vi "Digital Input Data.vi"(8 "error in (no error)":errorcluster, 10 "Digital Input Data":bool[](array[boolean]), 11 "Digital Reader in":refnum<class "Digital Reader.lvclass">) -> (0 "error out":errorcluster, 3 "Digital Reader out":refnum<class "Digital Reader.lvclass">)   [LabVIEW 2024, in "DAQmx Actor.lvlib" / "Digital Reader.lvclass"]
uses:
  Digital Reader.lvclass
  Digital Reader.lvclass/Digital Reader.ctl
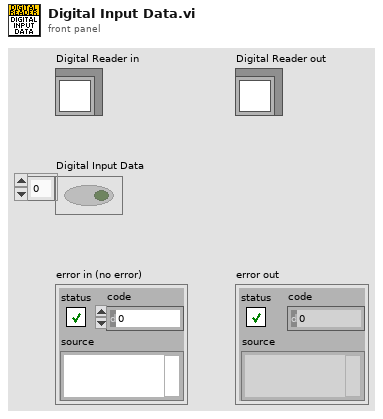
[diagram p1: front panel]
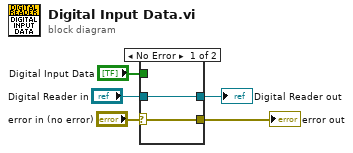
[diagram p0: block diagram]
diagram:
  n1 = case shown="No Error" "error in (no error)" {
    selector: "error in (no error)" -> [w6 w9]
    tunnel: [w6 w9] -> w4
    tunnel: [w7 w8] -> w2
    tunnel: "Digital Reader in" -> [w7 w8]
    tunnel: "Digital Input Data" -> [_ _]
    frame No Error {
    }
    frame Error {
    }
  }
  "error out" <- w4
  "Digital Reader out" <- w2
